vi "test for set multiple channels.vi"() -> ()   [LabVIEW 2013]
uses:
  <vilib>/NI Veristand/Execution/Workspace/NI_VS Workspace ExecutionAPI.lvlib
  Set Channels.lvlib
  <vilib>/NI Veristand/Execution/Workspace/NI VeriStand - Set Multiple Channel Values.vi
  <vilib>/NI Veristand/Execution/Workspace/NI VeriStand - Get Multiple Channel Values.vi
panel:
  out "Values":dbl[](array[numeric])
  in  "New Vals":dbl[](array[numeric]) format="%#_13g"
  in  "Array":string[](array[string])
  in  "Blocking?":bool
  out "error out":errorcluster
  out "Report Text":string
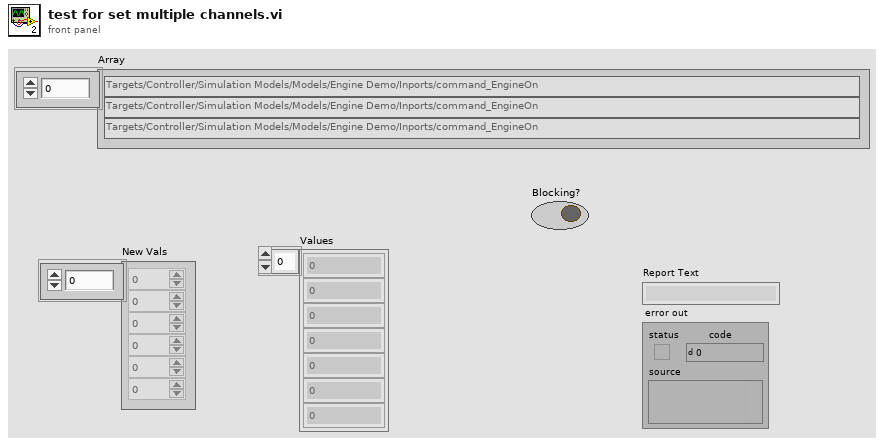
[diagram p1: front panel]
types:
  T1 = typedef "NI_VS Workspace ExecutionAPI.lvlib/WorkspaceAPI.ctl" = refnum<k24>
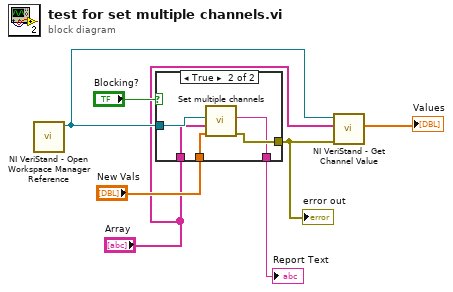
[diagram p0: block diagram]
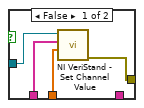
[diagram p2: hidden frame]
diagram:
  n1 = call <vilib>:"NI VeriStand - Open Workspace Manager Reference.vi"() -> ("WorkspaceManager"=w7:T1)  [unwired: 10 in, 1 out]
  n2 = case shown="True" "Blocking?" {
    tunnel: w7 -> [w11 w14]
    tunnel: [w10 w16] -> w6
    tunnel: [_ w15] -> w3
    tunnel: "Array" -> [w9 w13]
    tunnel: "New Vals" -> [w8 w12]
    frame False {
      n3 = call-poly <vilib>:"NI VeriStand - Set Channel Value.vi"("Values"=w8, "Channels"=w9, "WorkspaceManager in"=w11) -> ("error out"=w10:errorcluster)  [unwired: 7 in, 1 out]
    }
    frame True {
      n4 = call "Set multiple channels.vi"("values"=w12, "names"=w13, "Gateway IP Address (\"\": localhost)"=w14) -> ("error out"=w16:errorcluster, "Report Text"=w15:string)  [unwired: 6 in, 1 out]
    }
  }
  "Report Text" <- w3
  "error out" <- w6
  n5 = call-poly <vilib>:"NI VeriStand - Get Channel Value.vi"("error in (no error)"=w6, "Channels"="Array", "WorkspaceManager in"=w7) -> ("Values"=→"Values":dbl[])  [unwired: 6 in, 2 out]
